vi "Property Node (File Attributes).vi"   [LabVIEW 2020, in "NI_SFTP.lvlib"]
doc: "Gets (reads) or sets (writes) file attributes contained in a File Attributes object. These objects are returned by several SFTP functions, and can be used to update file attributes with the <b>Set File Attributes</b> function."
uses:
  <vilib>/net/SFTP/NI_SFTP.lvlib
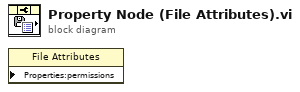
[diagram p0: block diagram]
diagram:
  n1 = property class="File Attributes" props=["Properties:permissions"]() -> ()  [unwired: 3 in, 2 out]
